vi "OMV_Snap.vi"(8 "error in (no error)":errorcluster, 11 "Python":T1) -> (0 "error out":errorcluster, 1 "picture":picture, 2 "image data":T3, 3 "Python":T1)   [LabVIEW 2020]
uses:
  <vilib>/picture/picture.llb/imagedata.ctl
  PythonCtrl.ctl
  Processors.ctl
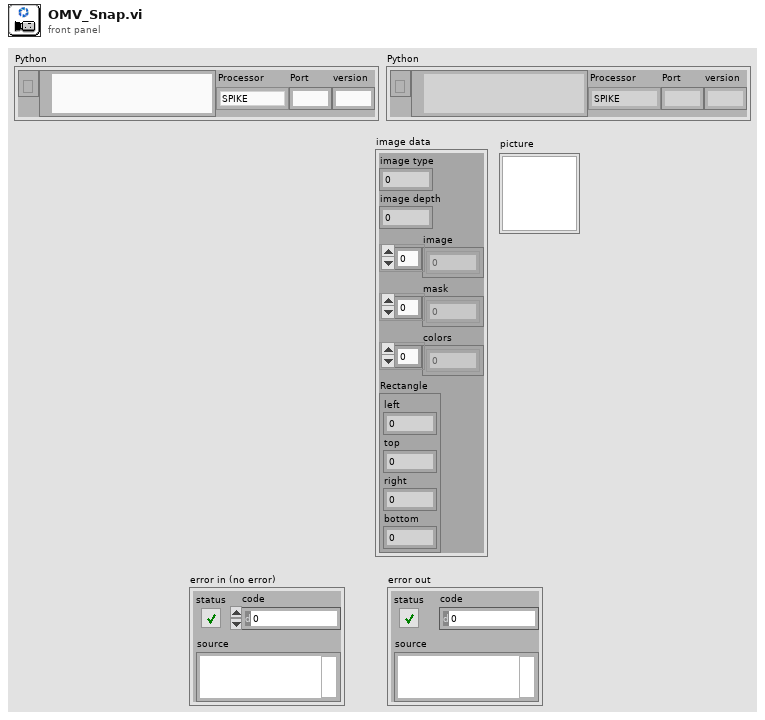
[diagram p1: front panel]
types:
  T1 = typedef "PythonCtrl.ctl" = cluster{"session":refnum<k35>, "PyPath":path, "Processor":T2, "Port":string, "version":string}
  T2 = typedef "Processors.ctl" = enum16{"SPIKE", "Pi", "Pi_ssh", "OpenMV", "Dunio"}
  T3 = typedef "imagedata.ctl" = cluster{"image type":i32, "image depth":i32, "image":u8[], "mask":u8[], "colors":u32[], "Rectangle":cluster{"left":i16, "top":i16, "right":i16, "bottom":i16}}
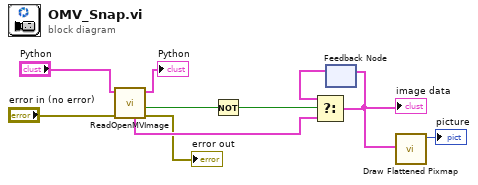
[diagram p0: block diagram]
diagram:
  n1 = call "ReadOpenMVImage.vi"("error in"="error in (no error)", "Python"="Python") -> ("error out"=→"error out":errorcluster, "Good?"=w6:bool, "Python"=→"Python":T1, "image data"=w8:T3)  [unwired: 4 in, 2 out]
  n2 = Not(x=w6) -> (.not. x?=w5:bool)
  n3 = feedback #1() -> (w7:T3)  [unwired: 1 in]
  n4 = Select(t=w7, s=w5, f=w8) -> (s? t:f=w4:T3)
  "image data" <- w4
  n5 = feedback-in #1(w4) -> ()
  n6 = call <vilib>:"Draw Flattened Pixmap.vi"("image data"=w4) -> ("new picture"=→"picture":picture)  [unwired: 8 in]
